vi "PosCtrl_Config_Threshold.vi"(4 "Negate Output":bool, 5 "Max Allowd Position":dbl=9e+30, 6 "At Reference Count":i32=13, 7 "Min Allowd Position":dbl=-9e+30, 8 "MinimumOutput":dbl=0.05, 9 "MaximumOutput":dbl=1.0, 10 "ErrorDeadband":dbl=0.08, 11 "ErrorThreshold":dbl=6.0) -> (3 "PosCtrl_Config_Params":T1={"Slope"=0.0, "Offset"=0.0, "Error Deadband"=0.0, "At Reference Count"=13, "Negate Output"=FALSE, "Max Allowd Position"=9e+30, "Min Allowd Position"=-9e+30})   [LabVIEW 2019, in "Trajectory_Library.lvlib"]
doc: "This VI creates the configuraation parameters for the position control controller. The straight line slope and intercept are calculated from the error threshold, error deadband, maximum output, and minimum output. A separate maximum output input to the controller executable allows the rate of output reduction to stey constant for different maximum output values. \n\nThe optional inputs Max Allowed Position and Min Allowed Position provide a virtual limit switch capability that forces the output to zero when it would cause movement in the direction of the exceeded limit.\n\nThe optional \"at refernce count\" parameter specifies the number of consecutive execution cycles the absolute value of the error has to be within the deadband to set \"At Reference\" to true. For a 20 millisecond loop time, the default value of 13 forces the error to be within the deadband for 260 milliseconds before At Reference is set to true.\n\nThe optional Negate Output parameter causes the output value to be multiplied by negative one.\n\nInputs:\n - Max Allowed Position - double - (Optional,, default: 9E+30 ) \n - Max Allowed Position - double - (Optional,, default: 9E+30 ) \n - Error threshold- double - When the error reaches this point, the output will start reducing from Maximum Output to Minimum output as the error decreases. Thie value must be positive.\n - Error Deadband - double - When the absolute value of the error is less than this, the output will be set to zero. Thie value must be positive.\n - Maximum Output - double - This is the output value used to calculate the slope of the slow down. The actual Maximum Output is specified in the Execute VI. The actual Maximum output can be greater or smaller than this value. Thie value must be positive.\n - Minimum Output - double - This is the output value when error reaches the Error Deadband. Thie value must be positive.\n - At Reference count - integer - The number of consecutive cycles that the error has to be within the Error Deadband to set the At Reference output to TRUE. (Optional, default: 13 )\n - Negate Output - boolean - When TRUE causes the output to be negated. (Optional, default: FALSE)\n\nOutputs:\n - PosCtrl_Config_Params - cluster - Data cluster containing the configuration parameters for the Position Control Execute VI."
uses:
  TypeDef/PosCtrl_Tuning_Type.ctl
  Trajectory_Library.lvlib
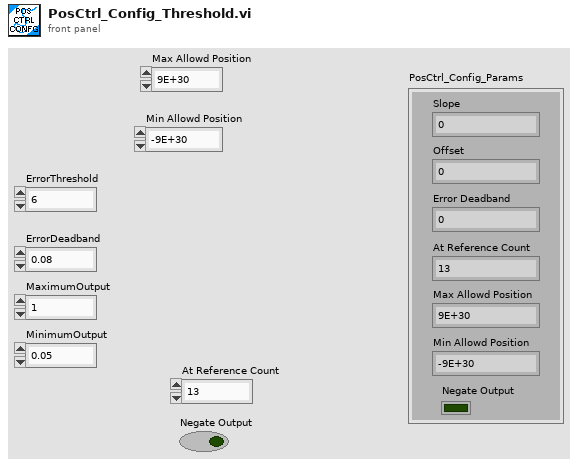
[diagram p1: front panel]
types:
  T1 = typedef "Trajectory_Library.lvlib/PosCtrl_Tuning_Type.ctl" = cluster{"Slope":dbl, "Offset":dbl, "Error Deadband":dbl, "At Reference Count":i32, "Negate Output":bool, "Max Allowd Position":dbl, "Min Allowd Position":dbl}
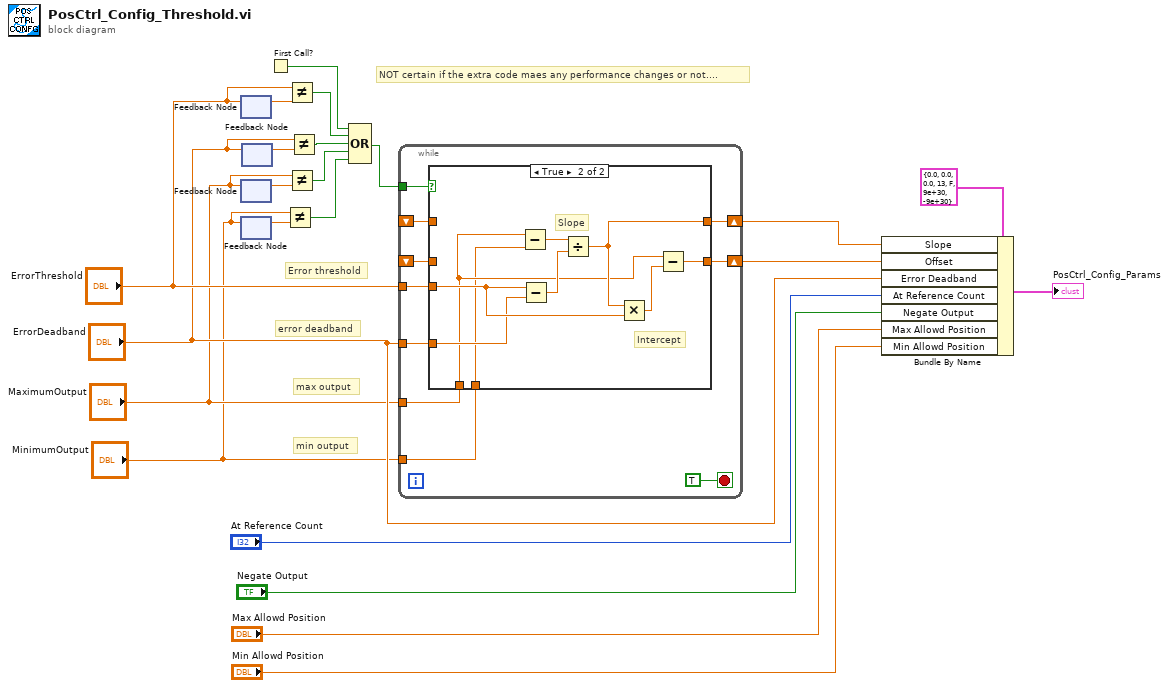
[diagram p0: block diagram]
diagram:
  # "NOT certain if the extra code maes any performance changes or not...."
  # "min output"
  # "Error threshold"
  # "error deadband"
  # "max output"
  n1 = feedback-in #1("ErrorThreshold") -> ()
  n2 = feedback #1() -> (w14:dbl)  [unwired: 1 in]
  n3 = feedback #2() -> (w10:dbl)  [unwired: 1 in]
  n4 = feedback-in #2("MaximumOutput") -> ()
  n5 = feedback #3() -> (w8:dbl)  [unwired: 1 in]
  n6 = feedback-in #3("MinimumOutput") -> ()
  n7 = feedback #4() -> (w12:dbl)  [unwired: 1 in]
  n8 = feedback-in #4("ErrorDeadband") -> ()
  n9 = First Call?() -> (First Call?: T/F=w2:bool)
  n10 = Not Equal?(x="MinimumOutput", y=w8) -> (x != y?=w3:bool)
  n11 = Not Equal?(x="ErrorThreshold", y=w14) -> (x != y?=w6:bool)
  n12 = Not Equal?(x="MaximumOutput", y=w10) -> (x != y?=w4:bool)
  n13 = Not Equal?(x="ErrorDeadband", y=w12) -> (x != y?=w5:bool)
  n14 = Compound Arithmetic op=OR(w2, w6, w5, w4, w3) -> (w1:bool)
  n15 = while {
    tunnel: "ErrorThreshold" -> [w30]
    tunnel: "ErrorDeadband" -> [w29]
    tunnel: "MaximumOutput" -> [w28]
    tunnel: "MinimumOutput" -> [w27]
    tunnel: w1 -> [w26]
    shift-right: [w32] -> w20
    shift-left: _ -> [w25]
    shift-right: [w31] -> w19
    shift-left: _ -> [w24]
    stop <- TRUE stop-if-true
    n16 = case shown="True" w26 {
      tunnel: [w34 w40] -> w32
      tunnel: [w33 w39] -> w31
      tunnel: w30 -> [_ w38]
      tunnel: w29 -> [_ w37]
      tunnel: w28 -> [_ w36]
      tunnel: w27 -> [_ w35]
      tunnel: w25 -> [w34 _]
      tunnel: w24 -> [w33 _]
      frame False {
      }
      frame True {
        # "Slope"
        # "Intercept"
        n17 = Subtract(x=w36, y=w35) -> (x-y=w41:dbl)
        n18 = Subtract(x=w38, y=w37) -> (x-y=w42:dbl)
        n19 = Divide(x=w41, y=w42) -> (x/y=w40:dbl)
        n20 = Multiply(x=w40, y=w38) -> (x*y=w43:dbl)
        n21 = Subtract(x=w36, y=w43) -> (x-y=w39:dbl)
      }
    }
  }
  n22 = Bundle By Name(cluster=T1 {"Slope"=0.0, "Offset"=0.0, "Error Deadband"=0.0, "At Reference Count"=13, "Negate Output"=FALSE, "Max Allowd Position"=9e+30, "Min Allowd Position"=-9e+30} ("PosCtrl_Config_Params"), "Slope"=w20, "Offset"=w19, "Error Deadband"="ErrorDeadband", "At Reference Count"="At Reference Count", "Negate Output"="Negate Output", "Max Allowd Position"="Max Allowd Position", "Min Allowd Position"="Min Allowd Position") -> (→"PosCtrl_Config_Params":T1)
